vi "Red Detection.vi"() -> ()   [LabVIEW 2018]
panel:
  out "Number of Matches (Detect red)":i32
  out "Number of Matches":i32
  out "Image overlay":T1(plugin-control)
  out "Frame Rate":dbl
  in  "stop":bool
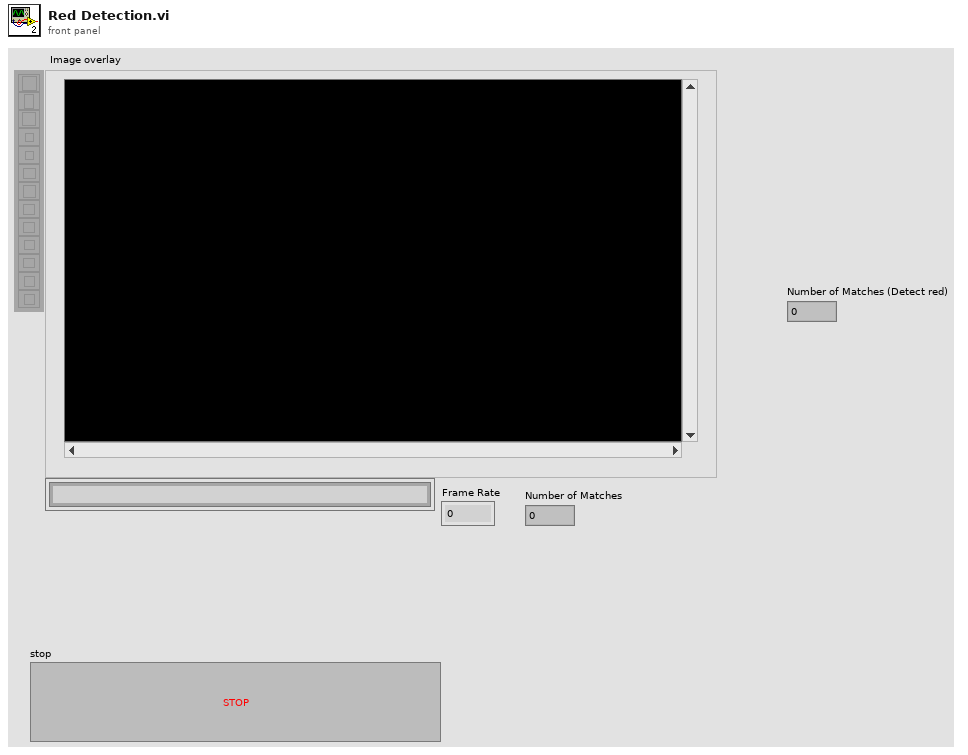
[diagram p1: front panel]
types:
  T1 = typedef "IMAQ Image.ctl" = refnum<image>
  T2 = cluster{"Desired Font (Application)":enum16{"User-specified Font", "Application Font", "System Font", "Dialog Font"}, "[User-specified Font]":cluster{"Font Name":string, "Size":i16, "Strikeout?":bool, "Italic?":bool, "Underline?":bool, "Outline?":bool, "Shadow?":bool, "Bold?":bool, "Rotation Angle":dbl}, "Horizontal Alignment":i16, "Vertical Alignment":i16}
  T3 = cluster{"Position":cluster{"x":sgl, "y":sgl}, "Angle":sgl, "Scale":sgl, "Score":sgl, "Bounding Box":cluster{"x":sgl, "y":sgl}[]}[]
  T4 = cluster{"Matches (Detect red)[0]":cluster{"Position":cluster{"x":sgl, "y":sgl}, "Angle":sgl, "Scale":sgl, "Score":sgl, "Bounding Box":cluster{"x":sgl, "y":sgl}[]}, "Matches (Detect red)[1]":cluster{"Position":cluster{"x":sgl, "y":sgl}, "Angle":sgl, "Scale":sgl, "Score":sgl, "Bounding Box":cluster{"x":sgl, "y":sgl}[]}, "Matches (Detect red)[2]":cluster{"Position":cluster{"x":sgl, "y":sgl}, "Angle":sgl, "Scale":sgl, "Score":sgl, "Bounding Box":cluster{"x":sgl, "y":sgl}[]}, "Matches (Detect red)[3]":cluster{"Position":cluster{"x":sgl, "y":sgl}, "Angle":sgl, "Scale":sgl, "Score":sgl, "Bounding Box":cluster{"x":sgl, "y":sgl}[]}, "Matches (Detect red)[4]":cluster{"Position":cluster{"x":sgl, "y":sgl}, "Angle":sgl, "Scale":sgl, "Score":sgl, "Bounding Box":cluster{"x":sgl, "y":sgl}[]}, "Matches (Detect red)[5]":cluster{"Position":cluster{"x":sgl, "y":sgl}, "Angle":sgl, "Scale":sgl, "Score":sgl, "Bounding Box":cluster{"x":sgl, "y":sgl}[]}, "Matches (Detect red)[6]":cluster{"Position":cluster{"x":sgl, "y":sgl}, "Angle":sgl, "Scale":sgl, "Score":sgl, "Bounding Box":cluster{"x":sgl, "y":sgl}[]}, "Matches (Detect red)[7]":cluster{"Position":cluster{"x":sgl, "y":sgl}, "Angle":sgl, "Scale":sgl, "Score":sgl, "Bounding Box":cluster{"x":sgl, "y":sgl}[]}, "Matches (Detect red)[8]":cluster{"Position":cluster{"x":sgl, "y":sgl}, "Angle":sgl, "Scale":sgl, "Score":sgl, "Bounding Box":cluster{"x":sgl, "y":sgl}[]}}
  T5 = cluster{"Bounding Box[0]":cluster{"x":sgl, "y":sgl}, "Bounding Box[1]":cluster{"x":sgl, "y":sgl}, "Bounding Box[2]":cluster{"x":sgl, "y":sgl}, "Bounding Box[3]":cluster{"x":sgl, "y":sgl}, "Bounding Box[4]":cluster{"x":sgl, "y":sgl}, "Bounding Box[5]":cluster{"x":sgl, "y":sgl}, "Bounding Box[6]":cluster{"x":sgl, "y":sgl}, "Bounding Box[7]":cluster{"x":sgl, "y":sgl}, "Bounding Box[8]":cluster{"x":sgl, "y":sgl}}
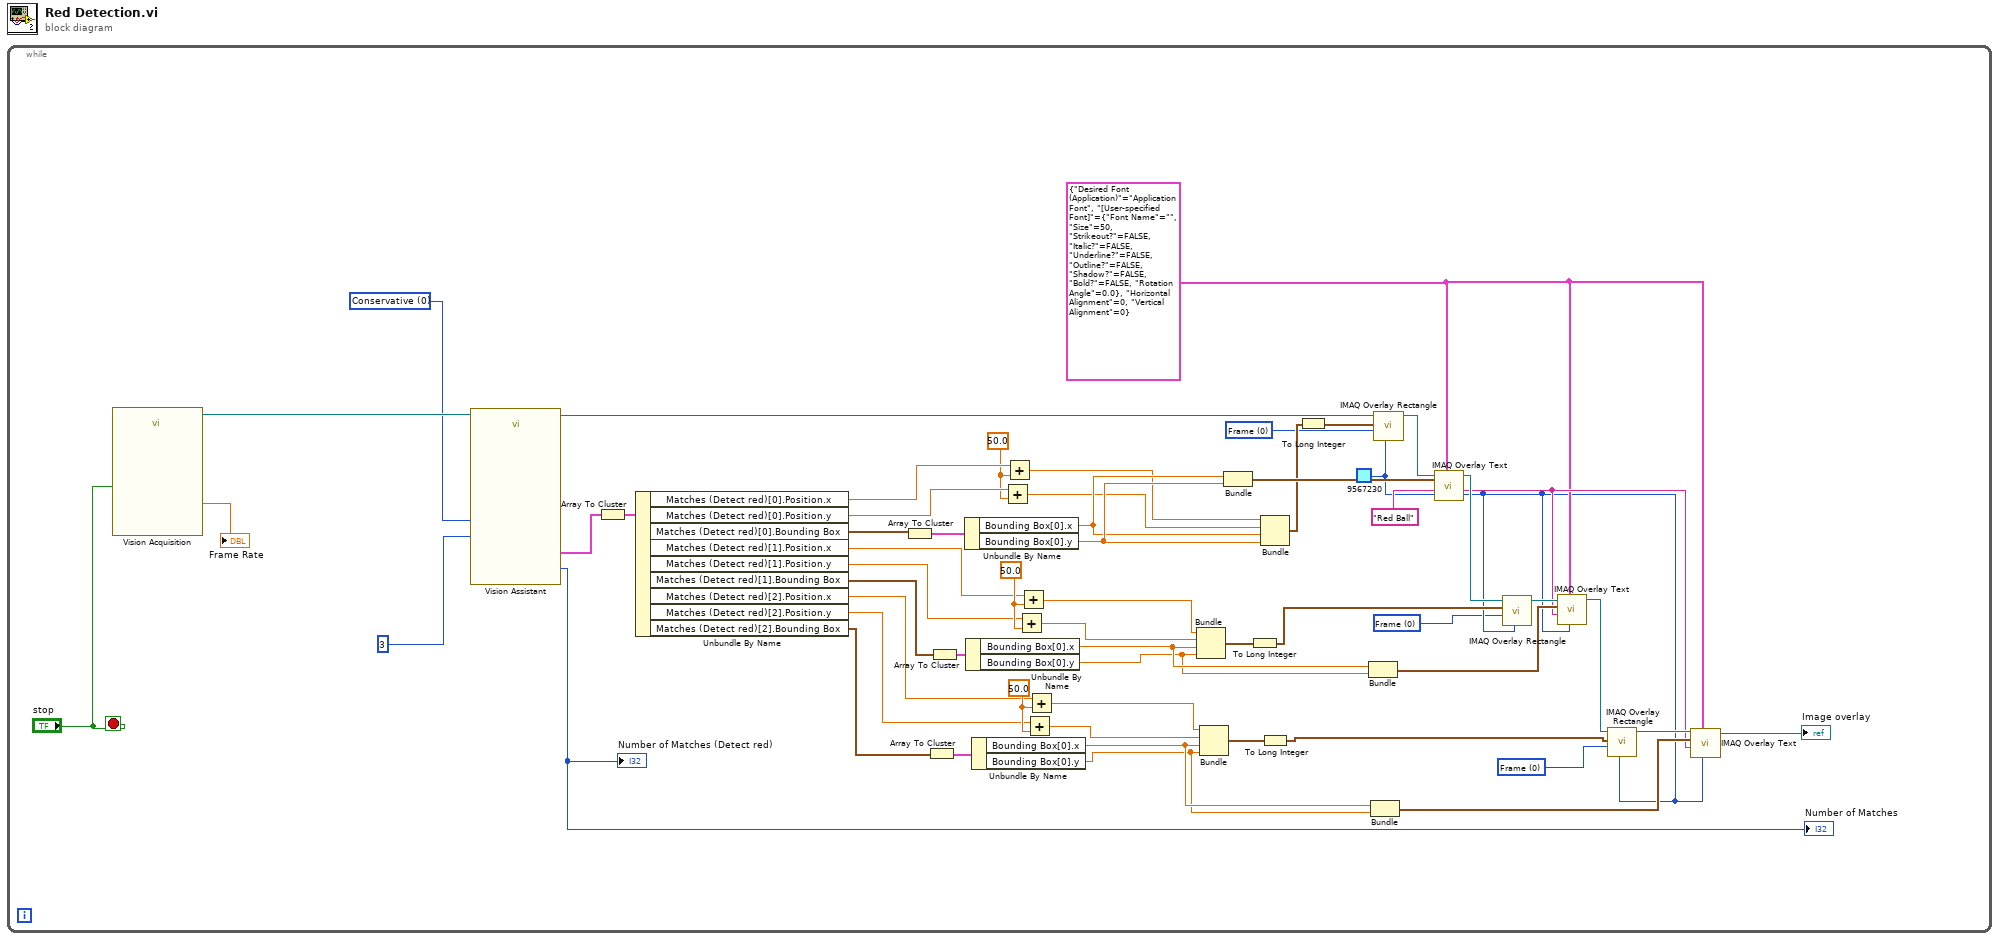
[diagram p0: block diagram]
diagram:
  n1 = while {
    stop <- "stop" stop-if-true
    w37 = u32 0 items=["Conservative", "Balance", "Aggressive", "Very Aggressive"] ("Search Strategy (Detect red)")
    w1 = u32 0 items=["Frame", "Fill", "Highlight"] ("Drawing Mode (Frame)")
    w9 = u32 0 items=["Frame", "Fill", "Highlight"] ("Drawing Mode (Frame)")
    w17 = sgl 50.0 ("y")
    w32 = sgl 50.0 ("y")
    w33 = sgl 50.0 ("y")
    w2 = u32 9567230 ("Text Color (black)")
    w3 = T2 {"Desired Font (Application)"=enum."Application Font", "[User-specified Font]"={"Font Name"="", "Size"=50, "Strikeout?"=FALSE, "Italic?"=FALSE, "Underline?"=FALSE, "Outline?"=FALSE, "Shadow?"=FALSE, "Bold?"=FALSE, "Rotation Angle"=0.0}, "Horizontal Alignment"=0, "Vertical Alignment"=0} ("Font, Size & Style")
    w4 = "Red Ball" ("String")
    w25 = u32 0 items=["Frame", "Fill", "Highlight"] ("Drawing Mode (Frame)")
    n2 = call "Vision Acquisition"("Stop (F)"="stop") -> ("Image Out"=w57:T1, "Frame Rate"=→"Frame Rate":dbl)  [unwired: 23 in, 2 out]
    n3 = call "Vision Assistant"("Image In"=w57, "Search Strategy (Detect red)"=w37, "Number of Matches Requested (Detect red)"=3) -> ("Image Out"=w50:T1, "Matches (Detect red)"=w52:T3, "Number of Matches (Detect red)"=→"Number of Matches" →"Number of Matches (Detect red)":i32)  [unwired: 21 in, 1 out]
    n4 = Array To Cluster(array=w52) -> (cluster=w51:T4)
    n5 = Unbundle By Name(w51) -> ("Matches (Detect red)[0].Position.x"=w41:sgl, "Matches (Detect red)[0].Position.y"=w39:sgl, "Matches (Detect red)[0].Bounding Box"=w49:cluster{"x":sgl, "y":sgl}[], "Matches (Detect red)[1].Position.x"=w31:sgl, "Matches (Detect red)[1].Position.y"=w30:sgl, "Matches (Detect red)[1].Bounding Box"=w35:cluster{"x":sgl, "y":sgl}[], "Matches (Detect red)[2].Position.x"=w16:sgl, "Matches (Detect red)[2].Position.y"=w15:sgl, "Matches (Detect red)[2].Bounding Box"=w18:cluster{"x":sgl, "y":sgl}[])
    n6 = Array To Cluster(array=w49) -> (cluster=w48:T5)
    n7 = Array To Cluster(array=w18) -> (cluster=w19:T5)
    n8 = Array To Cluster(array=w35) -> (cluster=w34:T5)
    n9 = Unbundle By Name(w48) -> ("Bounding Box[0].x"=w42:sgl, "Bounding Box[0].y"=w45:sgl)
    n10 = Unbundle By Name(w34) -> ("Bounding Box[0].x"=w22:sgl, "Bounding Box[0].y"=w21:sgl)
    n11 = Unbundle By Name(w19) -> ("Bounding Box[0].x"=w11:sgl, "Bounding Box[0].y"=w10:sgl)
    n12 = Add(x=w39, y=w33) -> (x+y=w38:sgl)
    n13 = Add(x=w41, y=w33) -> (x+y=w40:sgl)
    n14 = Add(x=w30, y=w32) -> (x+y=w28:sgl)
    n15 = Add(x=w31, y=w32) -> (x+y=w29:sgl)
    n16 = Add(x=w15, y=w17) -> (x+y=w13:sgl)
    n17 = Add(x=w16, y=w17) -> (x+y=w14:sgl)
    n18 = Bundle(w29, w28, "x"=w22, "y"=w21) -> (w27:cluster{sgl, sgl, "x":sgl, "y":sgl})  [unwired: 1 in]
    n19 = Bundle(w14, w13, "x"=w11, "y"=w10) -> (w12:cluster{sgl, sgl, "x":sgl, "y":sgl})  [unwired: 1 in]
    n20 = Bundle("x"=w42, "y"=w45) -> (w46:cluster{"x":sgl, "y":sgl})  [unwired: 1 in]
    n21 = To Long Integer(number=w27) -> (32bit integer=w26:cluster{i32, i32, "x":i32, "y":i32})
    n22 = Bundle(w40, w38, "x"=w42, "y"=w45) -> (w44:cluster{sgl, sgl, "x":sgl, "y":sgl})  [unwired: 1 in]
    n23 = To Long Integer(number=w12) -> (32bit integer=w7:cluster{i32, i32, "x":i32, "y":i32})
    n24 = To Long Integer(number=w44) -> (32bit integer=w43:cluster{i32, i32, "x":i32, "y":i32})
    n25 = Bundle("x"=w22, "y"=w21) -> (w20:cluster{"x":sgl, "y":sgl})  [unwired: 1 in]
    n26 = Bundle("x"=w11, "y"=w10) -> (w5:cluster{"x":sgl, "y":sgl})  [unwired: 1 in]
    n27 = call "IMAQ Overlay Rectangle"("Color"=w2, "Drawing Mode (Frame)"=w25, "Rectangle"=w43, "Image"=w50) -> ("Image Out"=w47:T1)  [unwired: 6 in, 1 out]
    n28 = call "IMAQ Overlay Text"("Text Color (black)"=w2, "Font, Size & Style"=w3, "String"=w4, "Origin"=w46, "Image"=w47) -> ("Image Out"=w23:T1)  [unwired: 5 in, 1 out]
    n29 = call "IMAQ Overlay Rectangle"("Color"=w2, "Drawing Mode (Frame)"=w1, "Rectangle"=w26, "Image"=w23) -> ("Image Out"=w24:T1)  [unwired: 6 in, 1 out]
    n30 = call "IMAQ Overlay Text"("Text Color (black)"=w2, "Font, Size & Style"=w3, "String"=w4, "Origin"=w20, "Image"=w24) -> ("Image Out"=w8:T1)  [unwired: 5 in, 1 out]
    n31 = call "IMAQ Overlay Rectangle"("Color"=w2, "Drawing Mode (Frame)"=w9, "Rectangle"=w7, "Image"=w8) -> ("Image Out"=w6:T1)  [unwired: 6 in, 1 out]
    n32 = call "IMAQ Overlay Text"("Text Color (black)"=w2, "Font, Size & Style"=w3, "String"=w4, "Origin"=w5, "Image"=w6) -> ("Image Out"=→"Image overlay":T1)  [unwired: 5 in, 1 out]
  }
